vi "On Idle.vi"(8 "error in (no error)":errorcluster, 11 "WebSocket in":refnum<class "WebSocket.lvclass">) -> (0 "error out":errorcluster, 3 "WebSocket out":refnum<class "WebSocket.lvclass">)   [LabVIEW 2023, in "WebSocket.lvclass"]
uses:
  WebSocket.lvclass
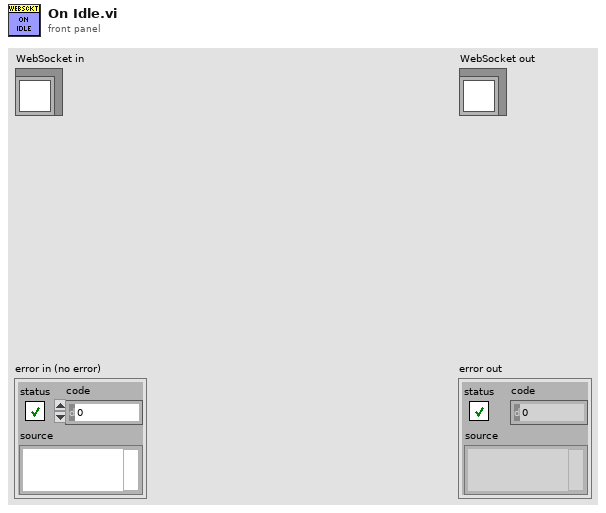
[diagram p1: front panel]
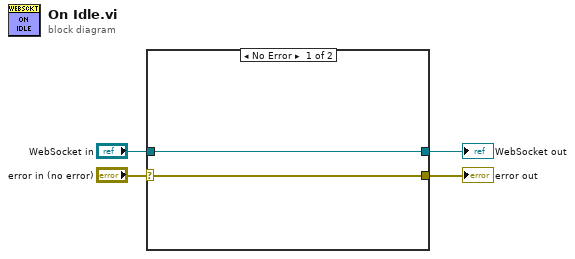
[diagram p0: block diagram]
diagram:
  n1 = case shown="No Error" "error in (no error)" {
    selector: "error in (no error)" -> [w5 w8]
    tunnel: [w5 w8] -> w3
    tunnel: [w6 w7] -> w1
    tunnel: "WebSocket in" -> [w6 w7]
    frame No Error {
    }
    frame Error {
    }
  }
  "error out" <- w3
  "WebSocket out" <- w1
